vi "Move Fwd PID.vi"(0 "Distance":dbl, 1 "Range":cluster{"output high":dbl, "output low":dbl}={"output high"=1.0, "output low"=0.0} {"output low" format="%.2f"; "output high" format="%.2f"}, 3 "Gains":T1={"proportional gain (Kc)"=1.0, "integral time (Ti, min)"=0.01, "derivative time (Td, min)"=0.0} {"derivative time (Td, min)" format="%.3f"; "integral time (Ti, min)" format="%.3f"; "proportional gain (Kc)" format="%.3f"}, 5 "Encoder Count":dbl, 7 "Reset Rate":bool, 9 "Time to stop":i32=300, 11 "Precision":dbl=0.5 format="%#_13g", 12 "Soft start":dbl=1.0, 14 "Loop Timer":i32=20) -> (4 "Finished?":bool, 15 "Output":dbl)   [LabVIEW 2020]
panel:
  in  "Integral Range":dbl=10000.0
  out "Waveform Chart":cluster{"Distance":dbl, "Encoder Count":dbl}(graph)
  # "Time to stop - Tempo que o encoder deve retornar um valor dentro do range da precision para a função considerar que o sistema está parado.\n\nDistance - Setpoint em unidades do encoder.\n\nLoop Timer - Tempo de iteração do loop em que a função está.\n\nPrecision - Range que a função considera \"close enough\" ao setpoint.\n\nEncoder Count - Valor atual do encoder.\n\nRate limit - Limite de aceleração/desaceleração do sistema.\n\nGains - Ganhos do PID.\n\nRange - limite superior e inferior do PID.\n\nSoft Start - constante que aumenta ou diminui o tempo de aceleração no início do movimento"
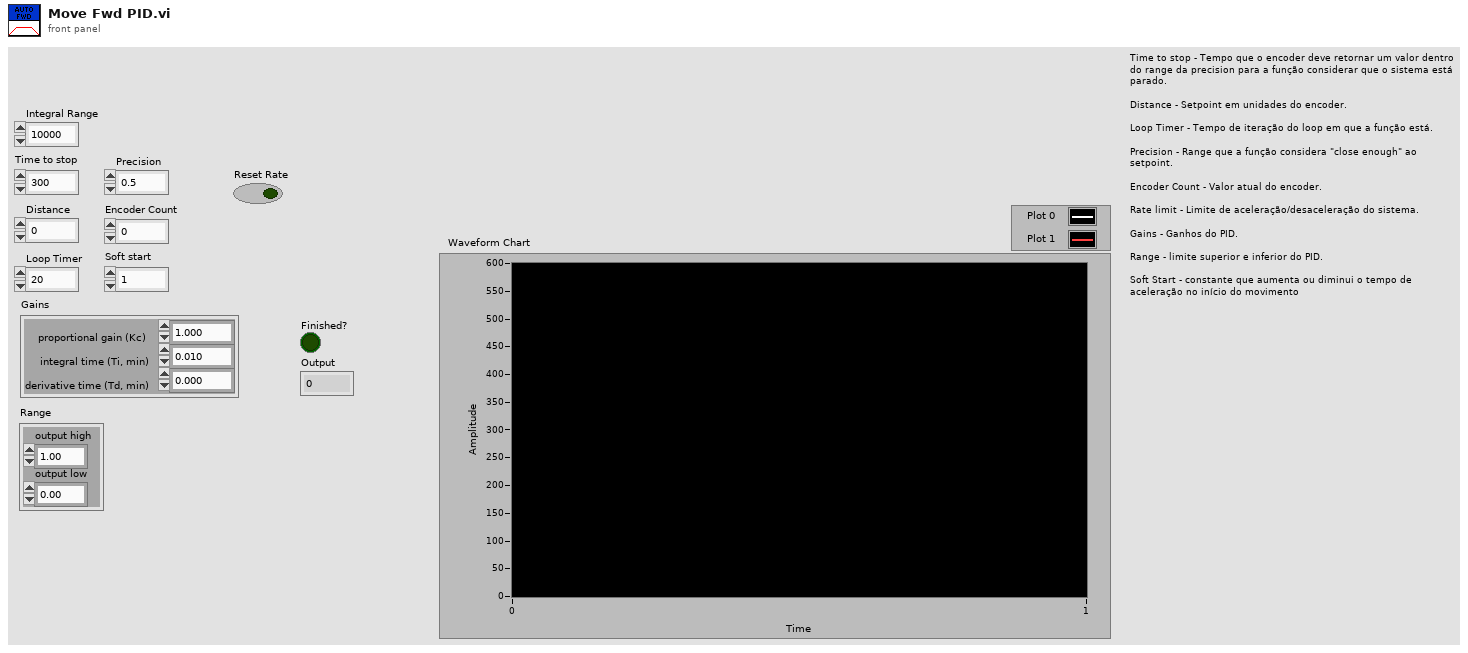
[diagram p1: front panel]
types:
  T1 = cluster{"proportional gain (Kc)":dbl, "integral time (Ti, min)":dbl, "derivative time (Td, min)":dbl}
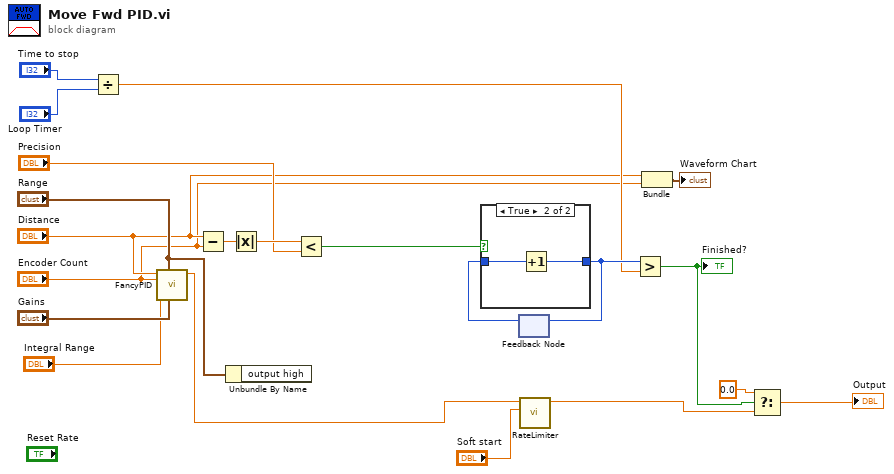
[diagram p0: block diagram]
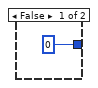
[diagram p2: hidden frame]
diagram:
  n1 = Divide(x="Time to stop", y="Loop Timer") -> (x/y=w15:dbl)
  n2 = call "FancyPID.vi"("Gains"="Gains", "Range"="Range", "Integral Range"="Integral Range", "Process variable"="Encoder Count", "Setpoint"="Distance") -> ("output"=w10:dbl)  [unwired: 6 in]
  n3 = Subtract(x="Distance", y="Encoder Count") -> (x-y=w14:dbl)
  n4 = Unbundle By Name("Range") -> ()  [unwired: 1 out]
  n5 = Absolute Value(x=w14) -> (abs(x)=w20:dbl)
  n6 = Less?(x=w20, y="Precision") -> (x < y?=w18:bool)
  n7 = feedback #1() -> (w17:i32)  [unwired: 1 in]
  n8 = case shown="True" w18 {
    tunnel: [0 w24] -> w16
    tunnel: w17 -> [_ w23]
    frame False {
    }
    frame True {
      n9 = Increment(x=w23) -> (x+1=w24:i32)
    }
  }
  n10 = feedback-in #1(w16) -> ()
  n11 = call "RateLimiter.vi"("Max dx/dt"="Soft start", "Input"=w10) -> ("Output"=w9:dbl)  [unwired: 9 in]
  n12 = Greater?(x=w16, y=w15) -> (0:w6:bool)
  "Finished?" <- w6
  n13 = Bundle("Distance"="Distance", "Encoder Count"="Encoder Count") -> (→"Waveform Chart":cluster{"Distance":dbl, "Encoder Count":dbl})  [unwired: 1 in]
  n14 = Select(t=0.0, s=w6, f=w9) -> (s? t:f=→"Output":dbl)
